vi "QueryServer_SetResponse_Invoke.vi"(0 "gRPCid":T1, 2 "status":i32, 3 "error in (no error)":errorcluster) -> (10 "error out":errorcluster)   [LabVIEW 2019, in "labview-grpc-query-server.lvlib"]
uses:
  labview-grpc-query-server.lvlib
  gRPC interface/Server API/typeDefs/grpcId.ctl
  QueryServer_InvokeResponse.ctl
  1048efad-fac4-412f-a2f0-e7e46cc14699.vi
  <vilib>/Utility/error.llb/Error Cluster From Error Code.vi
  gRPC interface/gprc-lvsupport.lvlib
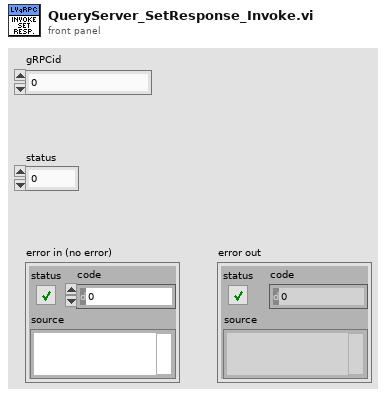
[diagram p1: front panel]
types:
  T1 = typedef "gprc-lvsupport.lvlib/grpcId.ctl" = u64
  T2 = typedef "labview-grpc-query-server.lvlib/QueryServer_InvokeResponse.ctl" = cluster{"status":i32}
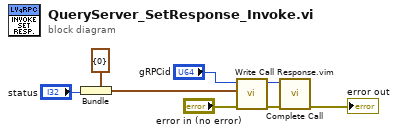
[diagram p0: block diagram]
diagram:
  n1 = Bundle(cluster=T2 {"status"=0} ("InvokeResponse"), "status"="status") -> (w5:T2)
  n2 = call "Write Call Response.vim"("error in (no error)"="error in (no error)", "Response Data"=w5, "gRPCid in"="gRPCid") -> ("error out"=w2:errorcluster, "gRPCid"=w3:T1)  [unwired: 7 in]
  n3 = call "Complete Call.vi"("gRPCid"=w3, "error in (no error)"=w2) -> ("error out"=→"error out":errorcluster)  [unwired: 8 in]
